vi "plot_counter_data_2.vi"(8 "error in (no error)":errorcluster, 10 "counter data 2":u32[][](array[numeric]), 11 "Cluster":T1) -> (0 "error out":errorcluster)   [LabVIEW 2011]
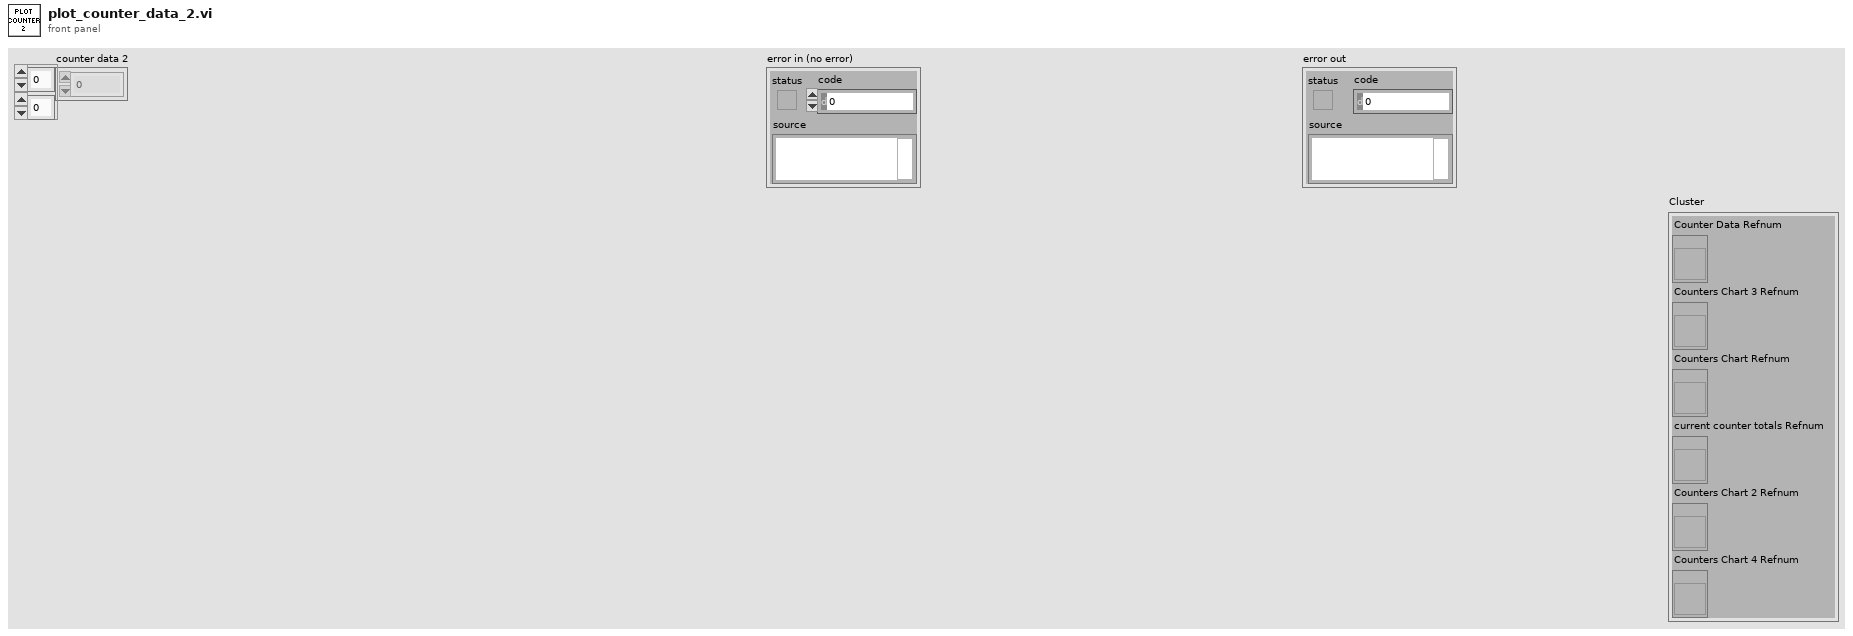
[diagram p1: front panel]
types:
  T1 = cluster{"Counter Data Refnum":refnum<vi>, "Counters Chart 3 Refnum":refnum<vi>, "Counters Chart Refnum":refnum<vi>, "current counter totals Refnum":refnum<vi>, "Counters Chart 2 Refnum":refnum<vi>, "Counters Chart 4 Refnum":refnum<vi>}
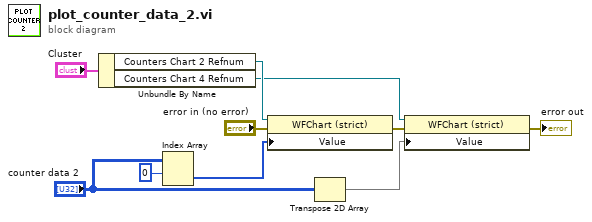
[diagram p0: block diagram]
diagram:
  n1 = Unbundle By Name("Cluster") -> ("Counters Chart 2 Refnum"=w9:refnum<vi>, "Counters Chart 4 Refnum"=w8:refnum<vi>)
  n2 = Index Array(array="counter data 2", index (row)=0) -> (element=w3:u32[])  [unwired: 1 in]
  n3 = property class="WFChart (strict)"(reference=w9, error in="error in (no error)", "Value"=w3) -> (error out=w7:errorcluster)  [unwired: 1 out]
  n4 = Transpose 2D Array(2D array="counter data 2") -> (transposed array=w2:u32[][])
  n5 = property class="WFChart (strict)"(reference=w8, error in=w7, "Value"=w2) -> (error out=→"error out":errorcluster)  [unwired: 1 out]
